vi "Move image.vi"(8 "Image Data":T6, 9 "Movement Data":T5) -> (2 "Image Data":T6)   [LabVIEW 2018]
doc: "Moves the logo on the stage based on the movement direction and increment."
uses:
  <vilib>/picture/picture.llb/imagedata.ctl
  Controls/DVD Data items/Movement Direction - Horizontal.ctl
  Controls/DVD Data items/Movement Direction - Vertical.ctl
  Controls/DVD Data items/Movement Increment (pix).ctl
  Controls/DVD Data items/Time Delay (ms).ctl
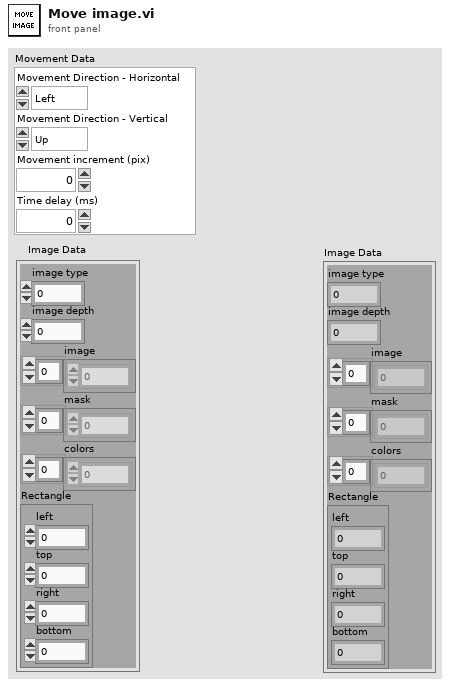
[diagram p1: front panel]
types:
  T1 = typedef "Movement Direction - Horizontal.ctl" = enum16{"Left", "Right"}
  T2 = typedef "Movement Direction - Vertical.ctl" = enum16{"Up", "Down"}
  T3 = typedef "Movement Increment (pix).ctl" = i16
  T4 = typedef "Time Delay (ms).ctl" = u8
  T5 = cluster{"Movement Direction - Horizontal":T1, "Movement Direction - Vertical":T2, "Movement increment (pix)":T3, "Time delay (ms)":T4}
  T6 = typedef "imagedata.ctl" = cluster{"image type":i32, "image depth":i32, "image":u8[], "mask":u8[], "colors":u32[], "Rectangle":cluster{"left":i16, "top":i16, "right":i16, "bottom":i16}}
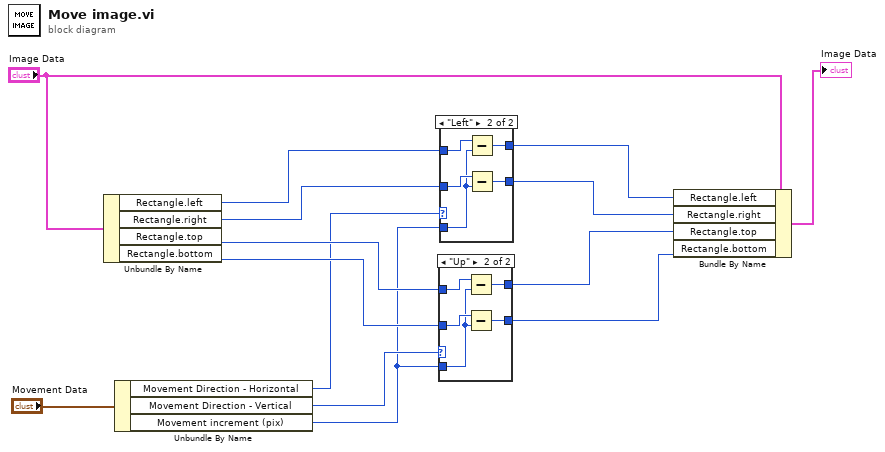
[diagram p0: block diagram]
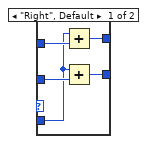
[diagram p2: hidden frame]
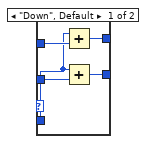
[diagram p3: hidden frame]
diagram:
  n1 = Unbundle By Name("Image Data") -> ("Rectangle.left"=w4:i16, "Rectangle.right"=w3:i16, "Rectangle.top"=w11:i16, "Rectangle.bottom"=w10:i16)
  n2 = Unbundle By Name("Movement Data") -> ("Movement Direction - Horizontal"=w6:T1, "Movement Direction - Vertical"=w7:T2, "Movement increment (pix)"=w5:T3)
  n3 = case shown="\"Up\"" w7 {
    tunnel: [w19 w24] -> w14
    tunnel: w11 -> [w18 w23]
    tunnel: w10 -> [w17 w22]
    tunnel: [w16 w21] -> w9
    tunnel: w5 -> [w15 w20]
    frame "Down", Default {
      n4 = Add(x=w15, y=w18) -> (x+y=w16:T3)
      n5 = Add(x=w15, y=w17) -> (x+y=w19:T3)
    }
    frame "Up" {
      n6 = Subtract(x=w23, y=w20) -> (x-y=w21:T3)
      n7 = Subtract(x=w22, y=w20) -> (x-y=w24:T3)
    }
  }
  n8 = case shown="\"Left\"" w6 {
    tunnel: [w29 w34] -> w1
    tunnel: w4 -> [w28 w33]
    tunnel: w3 -> [w27 w32]
    tunnel: [w26 w31] -> w2
    tunnel: w5 -> [w25 w30]
    frame "Right", Default {
      n9 = Add(x=w25, y=w28) -> (x+y=w26:T3)
      n10 = Add(x=w25, y=w27) -> (x+y=w29:T3)
    }
    frame "Left" {
      n11 = Subtract(x=w33, y=w30) -> (x-y=w31:T3)
      n12 = Subtract(x=w32, y=w30) -> (x-y=w34:T3)
    }
  }
  n13 = Bundle By Name(cluster="Image Data", "Rectangle.left"=w2, "Rectangle.right"=w1, "Rectangle.top"=w9, "Rectangle.bottom"=w14) -> (→"Image Data":T6)
